vi "test setting.vi"() -> ()   [LabVIEW 2013]
uses:
  VIs/ClientServerMode/CS_LFAClassGlobal.vi
  LightField Automation.lvclass
panel:
  out "ADCQuality":u16(ring)=4 items=["LowNoise"=1, "HighCapacity"=2, "ElectronMultiplied"=3, "HighSpeed"=4]
  in  "data 3":string
  in  "data":string
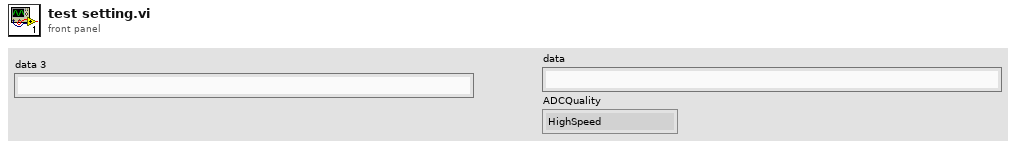
[diagram p1: front panel]
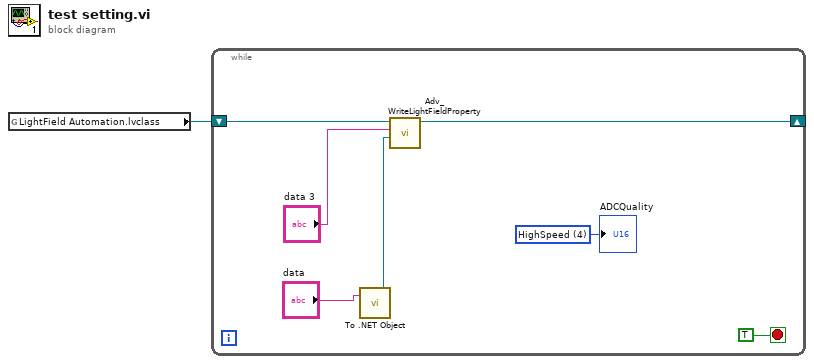
[diagram p0: block diagram]
diagram:
  n1 = global read "CS_LFAClassGlobal.vi" "LightField Automation.lvclass"() -> (w1:refnum<class "LightField Automation.lvclass">)
  n2 = while {
    shift-right: [w3] -> _
    shift-left: w1 -> [w7]
    stop <- TRUE stop-if-true
    w2 = u16 4 items=["LowNoise"=1, "HighCapacity"=2, "ElectronMultiplied"=3, "HighSpeed"=4] ("ADCQuality")
    n3 = call <vilib>:"To .NET Object.vi"("anything"="data") -> (".NET object"=w5:refnum<k24>)  [unwired: 1 in, 1 out]
    n4 = call "Adv_WriteLightFieldProperty.vi"("value"=w5, "setting"="data 3", "LightField Automation in"=w7) -> ("LightField Automation out"=w3:refnum<class "LightField Automation.lvclass">)  [unwired: 7 in, 1 out]
    "ADCQuality" <- w2
  }
